vi "Read Image Dimensions.vi"(8 "error in (no error)":errorcluster, 11 "CCDCamera in":refnum<class "Simulated_CCD_Camera.lvclass">) -> (0 "error out":errorcluster, 2 "CCD Config":T1={"Exposure Time"=1.0, "Pre-amp gain"=0, "Readout Rate"=0, "EM Mode"=0, "EM Gain"=2, "Binning"=1, "Initial Line"=1, "Initial Cloumn"=1, "Final Line"=1024, "Final Column"=1024, "Kinetic Series Length"=1, "Shutter Mode"=2, "Cooler ON/OFF"=0, "Temperature"=0, "Image Name"="CH1", "Image Path"="C:\\Users\\observer\\Desktop\\Imagens", "Current Temperature"=20, "Temperatue Status"="TEMPERATURE OFF", "Serial Number"=9916, " #image"=0} {"Temperature" min=0 max=0; "EM Mode" items=["Electron Multiplying", "Conventional"]; "Readout Rate" items=["1 MHz", "10 MHz", "20 MHz", "30 MHz"]; "Pre-amp gain" items=["Gain 1", "Gain 2"]}, 3 "CCDCamera out":refnum<class "Simulated_CCD_Camera.lvclass">)   [LabVIEW 2018, in "Simulated_CCD_Camera.lvclass"]
uses:
  Simulated_CCD_Camera.lvclass
  Simulated_Cooler/Simulated_Cooler.lvclass
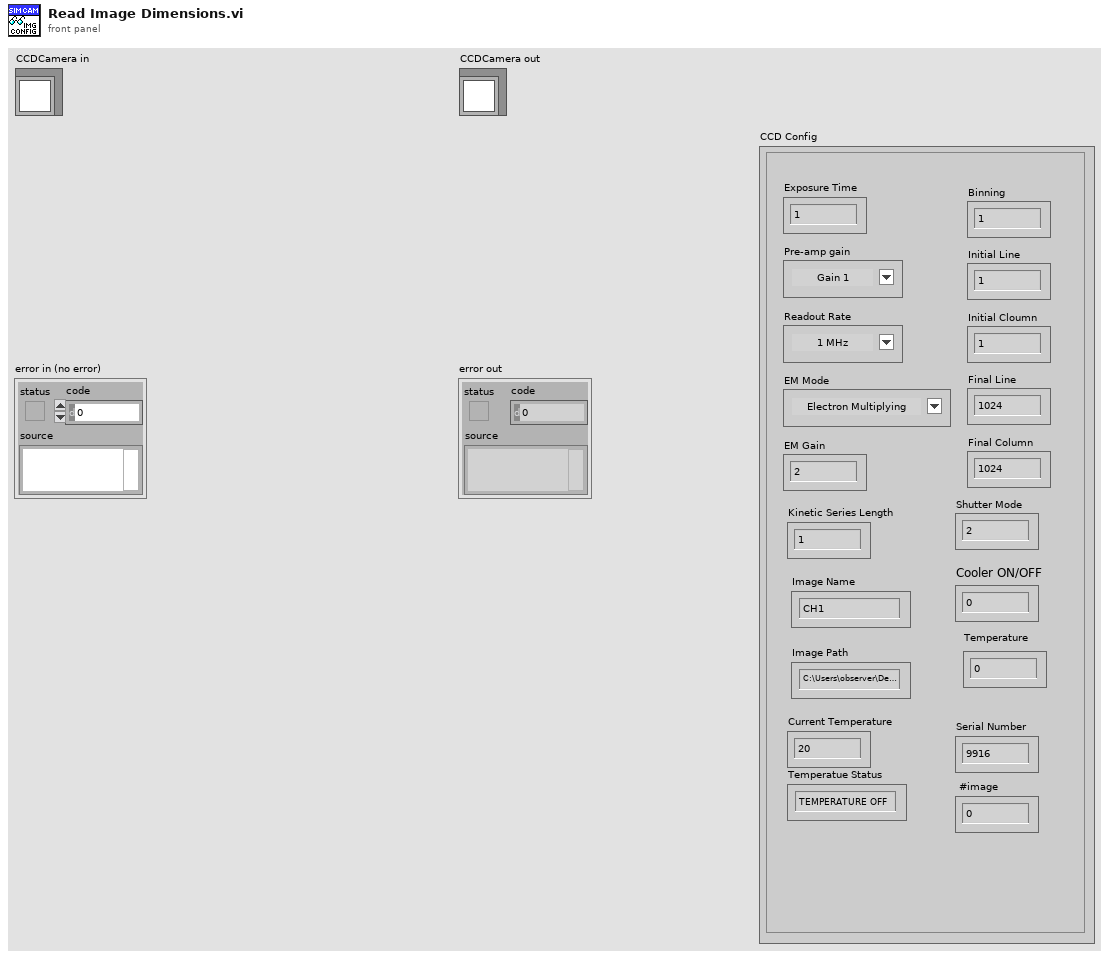
[diagram p1: front panel]
types:
  T1 = cluster{"Exposure Time":sgl, "Pre-amp gain":u8, "Readout Rate":u8, "EM Mode":u8, "EM Gain":u16, "Binning":u16, "Initial Line":u16, "Initial Cloumn":u16, "Final Line":u16, "Final Column":u16, "Kinetic Series Length":u32, "Shutter Mode":u8, "Cooler ON/OFF":u8, "Temperature":i8, "Image Name":string, "Image Path":string, "Current Temperature":i16, "Temperatue Status":string, "Serial Number":u16, " #image":u32}
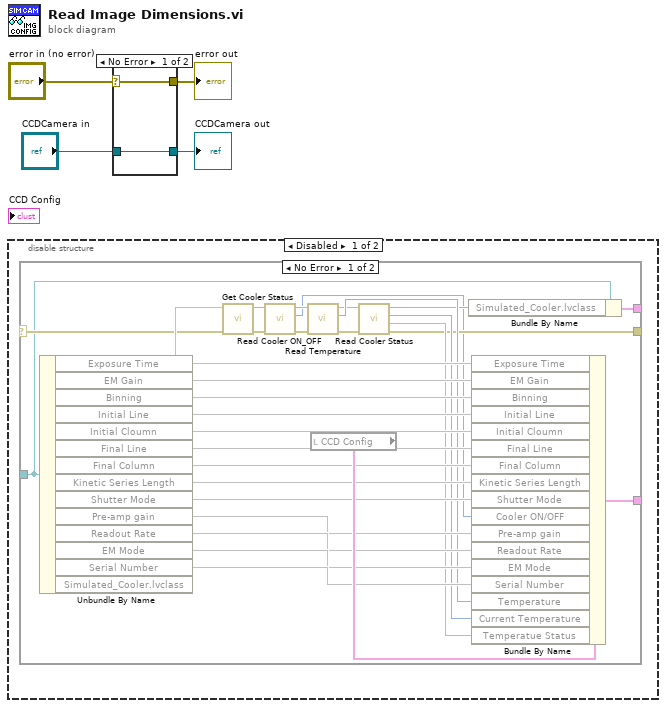
[diagram p0: block diagram]
diagram:
  n1 = disable-structure shown="Disabled" {
    frame Disabled {
      n2 = case shown="No Error" {
        selector: _ -> [w19 w37]
        tunnel: [w13 w37] -> _
        tunnel: [w10 w36] -> _
        tunnel: _ -> [w12 w36]
        tunnel: [w34 _] -> _
        frame No Error {
          n3 = Unbundle By Name(w12) -> ("Exposure Time"=w22, "EM Gain"=w23, "Binning"=w24, "Initial Line"=w25, "Initial Cloumn"=w26, "Final Line"=w27, "Final Column"=w28, "Kinetic Series Length"=w29, "Shutter Mode"=w21, "Pre-amp gain"=w30, "Readout Rate"=w31, "EM Mode"=w32, "Serial Number"=w33, "Simulated_Cooler.lvclass"=w20)
          n4 = call-dynamic "Get Cooler Status.vi"("error in (no error)"=w19, "Cooler in"=w20) -> ("error out"=w7:errorcluster, "Cooler out"=w8:refnum<class "Simulated_Cooler.lvclass">)  [unwired: 8 in]
          n5 = call "Read Cooler ON_OFF.vi"("error in (no error)"=w7, "Cooler in"=w8) -> ("error out"=w6:errorcluster, "Cooler ON/OFF"=w5:u8, "Cooler out"=w9:refnum<class "Simulated_Cooler.lvclass">)  [unwired: 7 in]
          n6 = call-dynamic "Read Temperature.vi"("error in (no error)"=w6, "Cooler in"=w9) -> ("error out"=w15:errorcluster, "Temperature"=w16:i32, "Cooler out"=w14:refnum<class "Simulated_Cooler.lvclass">)  [unwired: 7 in]
          n7 = local read "CCD Config"() -> (w35:T1)
          n8 = call "Read Cooler Status.vi"("error in (no error)"=w15, "Cooler in"=w14) -> ("error out"=w13:errorcluster, "temp status"=w17:string, "Current temp"=w18:i16, "Cooler out"=w11:refnum<class "Simulated_Cooler.lvclass">)  [unwired: 6 in]
          n9 = Bundle By Name(cluster=w12, "Simulated_Cooler.lvclass"=w11) -> (w10:cluster{})
          n10 = Bundle By Name(cluster=w35, "Exposure Time"=w22, "EM Gain"=w23, "Binning"=w24, "Initial Line"=w25, "Initial Cloumn"=w26, "Final Line"=w27, "Final Column"=w28, "Kinetic Series Length"=w29, "Shutter Mode"=w21, "Cooler ON/OFF"=w5, "Pre-amp gain"=w30, "Readout Rate"=w31, "EM Mode"=w32, "Serial Number"=w33, "Temperature"=w16, "Current Temperature"=w18, "Temperatue Status"=w17) -> (w34:T1)
        }
        frame Error {
        }
      }
    }
    frame Enabled {
    }
  }
  n11 = case shown="No Error" "error in (no error)" {
    selector: "error in (no error)" -> [w38 w41]
    tunnel: [w38 w41] -> w3
    tunnel: [w39 w40] -> w1
    tunnel: "CCDCamera in" -> [w39 w40]
    frame No Error {
    }
    frame Error {
    }
  }
  "error out" <- w3
  "CCDCamera out" <- w1
